vi "Log file.vi"(8 "error in (no error)":errorcluster) -> (0 "error in (no error) 2":errorcluster)   [LabVIEW 2018]
uses:
  <vilib>/addons/_JKI Toolkits/Caraya/classes/Test/Test.lvclass
  Log File/Log File.lvclass
  <vilib>/addons/_JKI Toolkits/Caraya/classes/Assert/Assert.lvclass
  <vilib>/addons/_JKI Toolkits/Caraya/classes/Assert/Assert Not Error.vi
  <vilib>/addons/_JKI Toolkits/Caraya/classes/Assert/Assert Equal Value_Variant.vi
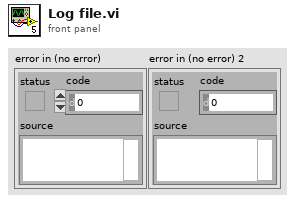
[diagram p1: front panel]
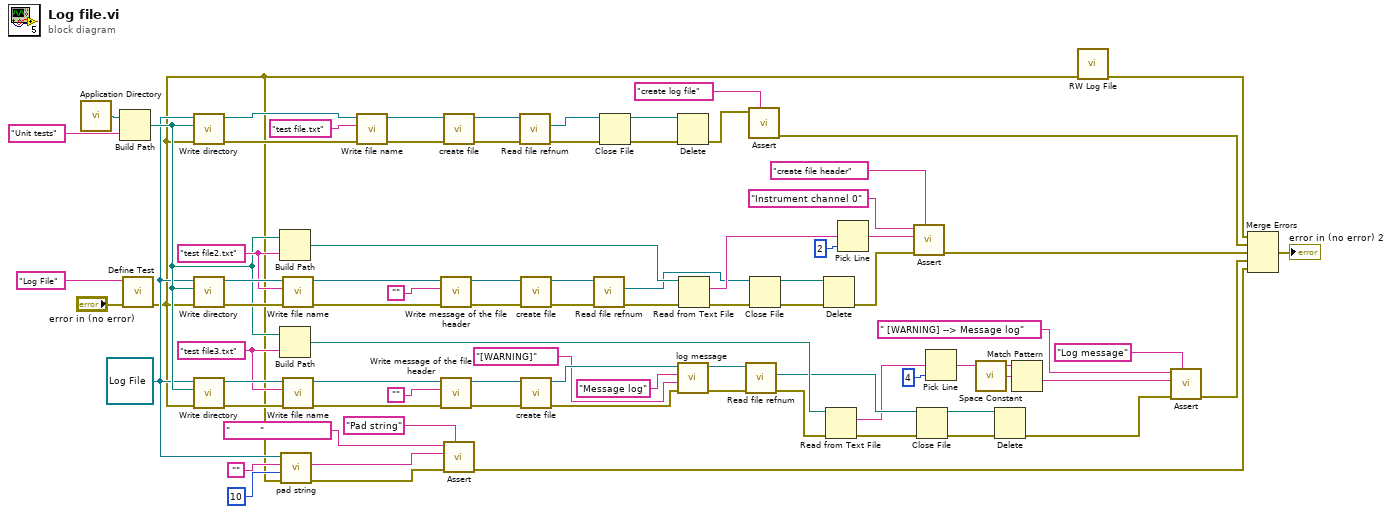
[diagram p0: block diagram]
diagram:
  w27 = "test file3.txt" ("file name")
  w53 = "test file2.txt" ("file name")
  w9 = refnum<class "Log File.lvclass"> refnum ("Log File in")
  n1 = call <vilib>:"Application Directory.vi"() -> ("Application Directory"=w76:path)
  n2 = Build Path(base path=w76, name or relative path="Unit tests") -> (appended path=w26:path)
  n3 = call <vilib>:"Define Test.vi"("error in (no error)"="error in (no error)", "Label (VI Title)"="Log File") -> ("error out"=w1:errorcluster)  [unwired: 8 in, 1 out]
  n4 = call "Write directory.vi"("error in (no error)"=w1, 10:w26, "Log File in"=w9) -> ("error out"=w78:errorcluster, "Log File out"=w77:refnum<class "Log File.lvclass">)  [unwired: 7 in]
  n5 = call "Write directory.vi"("error in (no error)"=w1, 10:w26, "Log File in"=w9) -> ("error out"=w62:errorcluster, "Log File out"=w61:refnum<class "Log File.lvclass">)  [unwired: 7 in]
  n6 = call "Write directory.vi"("error in (no error)"=w1, 10:w26, "Log File in"=w9) -> ("error out"=w37:errorcluster, "Log File out"=w36:refnum<class "Log File.lvclass">)  [unwired: 7 in]
  n7 = Build Path(base path=w26, name or relative path=w53) -> (appended path=w52:path)
  n8 = Build Path(base path=w26, name or relative path=w27) -> (appended path=w28:path)
  n9 = call "pad string.vi"("error in (no error)"=w1, "string size"=u16 10, "input string"="", "Log File in"=w9) -> ("error out"=w2:errorcluster, "output string"=w6:string)  [unwired: 5 in, 1 out]
  n10 = call "Write file name.vi"("error in (no error)"=w62, "suffix"=w53, "Log File in"=w61) -> ("error out"=w57:errorcluster, "Log File out"=w60:refnum<class "Log File.lvclass">)  [unwired: 7 in]
  n11 = call "Write file name.vi"("error in (no error)"=w37, "suffix"=w27, "Log File in"=w36) -> ("error out"=w40:errorcluster, "Log File out"=w35:refnum<class "Log File.lvclass">)  [unwired: 7 in]
  n12 = call "Write file name.vi"("error in (no error)"=w78, "suffix"="test file.txt" ("file name"), "Log File in"=w77) -> ("error out"=w63:errorcluster, "Log File out"=w64:refnum<class "Log File.lvclass">)  [unwired: 7 in]
  n13 = call "Write message of the file header.vi"("error in (no error)"=w57, "message of the file header"="", "Log File in"=w60) -> ("error out"=w58:errorcluster, "Log File out"=w59:refnum<class "Log File.lvclass">)  [unwired: 7 in]
  n14 = call "Write message of the file header.vi"("error in (no error)"=w40, "message of the file header"="", "Log File in"=w35) -> ("error out"=w39:errorcluster, "Log File out"=w34:refnum<class "Log File.lvclass">)  [unwired: 7 in]
  n15 = call "create file.vi"("error in (no error)"=w63, "Log File in"=w64) -> ("error out"=w66:errorcluster, "Log File out"=w65:refnum<class "Log File.lvclass">)  [unwired: 8 in]
  n16 = call-poly <vilib>:"Assert.vi"("Label"="Pad string" ("Label (VI Title)"), "error in (no error)"=w2, "Actual"=w6, "Expected"="          ") -> ("error out"=w3:errorcluster)  [unwired: 6 in, 1 out]
  n17 = call "Read file refnum.vi"("error in (no error)"=w66, "Log File in"=w65) -> ("error out"=w70:errorcluster, "file refnum"=w67:refnum<file>)  [unwired: 7 in, 1 out]
  n18 = call "create file.vi"("error in (no error)"=w58, "Log File in"=w59) -> ("error out"=w56:errorcluster, "Log File out"=w55:refnum<class "Log File.lvclass">)  [unwired: 8 in]
  n19 = call "create file.vi"("error in (no error)"=w39, "Log File in"=w34) -> ("error out"=w38:errorcluster, "Log File out"=w31:refnum<class "Log File.lvclass">)  [unwired: 8 in]
  n20 = call "Read file refnum.vi"("error in (no error)"=w56, "Log File in"=w55) -> ("error out"=w54:errorcluster, "file refnum"=w41:refnum<file>)  [unwired: 7 in, 1 out]
  n21 = Close File(refnum=w67, error in=w70) -> (path=w68:path, error out=w69:errorcluster)
  n22 = Delete(path (use dialog)=w68, error in=w69) -> (error out=w74:errorcluster)  [unwired: 3 in, 2 out]
  n23 = call-dynamic "log message.vi"("error in (no error)"=w38, "message type"="[WARNING]", "Message to log"="Message log", "Log File in"=w31) -> ("error out"=w17:errorcluster, "Log File out"=w16:refnum<class "Log File.lvclass">)  [unwired: 6 in]
  n24 = Read from Text File(file (use dialog)=w52, error in=w54) -> (text=w51:string, error out=w45:errorcluster)  [unwired: 2 in, 2 out]
  n25 = call "Read file refnum.vi"("error in (no error)"=w17, "Log File in"=w16) -> ("error out"=w15:errorcluster, "file refnum"=w14:refnum<file>)  [unwired: 7 in, 1 out]
  n26 = call-poly <vilib>:"Assert.vi"("Label"="create log file" ("Label (VI Title)"), "Not Error?"=w74) -> ("error out"=w73:errorcluster)  [unwired: 8 in, 1 out]
  n27 = Close File(refnum=w41, error in=w45) -> (path=w43:path, error out=w46:errorcluster)
  n28 = Delete(path (use dialog)=w43, error in=w46) -> (error out=w44:errorcluster)  [unwired: 3 in, 2 out]
  n29 = Read from Text File(file (use dialog)=w28, error in=w15) -> (text=w11:string, error out=w23:errorcluster)  [unwired: 2 in, 2 out]
  n30 = Pick Line(multi-line string=w51, line index=2) -> (output string=w49:string)  [unwired: 1 in]
  n31 = call-poly <vilib>:"Assert.vi"("Label"="create file header" ("Label (VI Title)"), "error in (no error)"=w44, "Actual"=w49, "Expected"="Instrument channel 0" ("Label (VI Title)")) -> ("error out"=w47:errorcluster)  [unwired: 6 in, 1 out]
  n32 = Close File(refnum=w14, error in=w23) -> (path=w25:path, error out=w24:errorcluster)
  n33 = Pick Line(multi-line string=w11, line index=4) -> (output string=w12:string)  [unwired: 1 in]
  n34 = call <vilib>:"Space Constant.vi"() -> ("String"=w18:string)
  n35 = Delete(path (use dialog)=w25, error in=w24) -> (error out=w21:errorcluster)  [unwired: 3 in, 2 out]
  n36 = Match Pattern(string=w12, regular expression=w18) -> (after substring=w19:string)  [unwired: 1 in, 3 out]
  n37 = call "RW Log File.vi"("error in (no error)"=w1) -> ("error in (no error) 2"=w79:errorcluster)  [unwired: 10 in]
  n38 = call-poly <vilib>:"Assert.vi"("Label"="Log message" ("Label (VI Title)"), "error in (no error)"=w21, "Actual"=w19, "Expected"=" [WARNING] --> Message log" ("Label (VI Title)")) -> ("error out"=w22:errorcluster)  [unwired: 6 in, 1 out]
  n39 = Merge Errors(w79, w73, w47, w22, w3) -> (→"error in (no error) 2":errorcluster)
